vi "CRYSelect curve by name.vi"(9 "Curve name desired (just name, if flat data not wired)":string, 10 "Curve name desired (flat data)":string, 11 "Data array":T2 {"Z data" items=["dB", "Lin"]; "X data" items=["dB", "Lin"]; "Y data" items=["dB", "Lin"]; "Z dB ref" format="%.1f"; "Z axis" items=["Log", "Lin"]; "X dB ref" format="%.1f"; "X axis" items=["Log", "Lin"]; "Y axis" items=["Log", "Lin"]; "Y dB ref" format="%.1f"; "Curve"."z" format="%.2f"; "Curve"."y" format="%.2f"; "Curve"."x" format="%.2f"}) -> (0 "Exists?":bool, 1 "Valid curve desired?":bool, 3 "Desired Curve":T1={"Name"="", "Curve"=[], "X data"=1, "Y data"=1, "Z data"=1, "X axis"=0, "Y axis"=1, "Z axis"=1, "X unit"="Hz", "Y unit"="", "Z unit"="deg.", "X dB ref"=1.0, "Y dB ref"=1.0, "Z dB ref"=1.0, "single val"=FALSE, "protected"=FALSE, "display X"=TRUE, "display Y"=TRUE, "display Z"=TRUE, "Test Info"="", "Step No."=0, "Plot Settings"={"Color"=0, "Interpolation"=0, "Point Style"=0, "Line Style"=0, "Point Color"=0, "Line Width"=0, "Bar Plot Style"=0, "Fill To"=0}, "AutoProtect"=FALSE} {"Z data" items=["dB", "Lin"]; "X data" items=["dB", "Lin"]; "Y data" items=["dB", "Lin"]; "Z dB ref" format="%.1f"; "Z axis" items=["Log", "Lin"]; "X dB ref" format="%.1f"; "X axis" items=["Log", "Lin"]; "Y axis" items=["Log", "Lin"]; "Y dB ref" format="%.1f"; "Curve"."z" format="%.2f"; "Curve"."y" format="%.2f"; "Curve"."x" format="%.2f"}, 5 "index of element":i32)   [LabVIEW 2013]
uses:
  Typedef Control/CRYData Cluster Array.ctl
  Typedef Control/CRYData Cluster.ctl
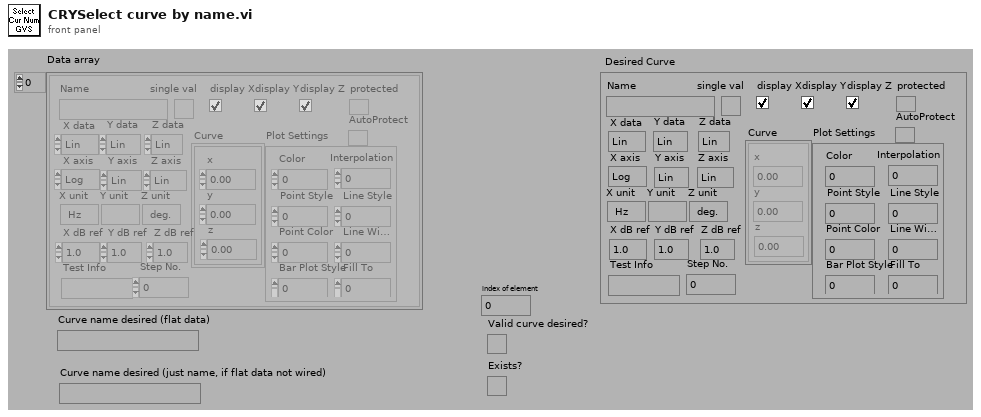
[diagram p1: front panel]
types:
  T1 = typedef "CRYData Cluster.ctl" = cluster{"Name":string, "Curve":cluster{"x":dbl, "y":dbl, "z":dbl}[], "X data":u16, "Y data":u16, "Z data":u16, "X axis":u16, "Y axis":u16, "Z axis":u16, "X unit":string, "Y unit":string, "Z unit":string, "X dB ref":dbl, "Y dB ref":dbl, "Z dB ref":dbl, "single val":bool, "protected":bool, "display X":bool, "display Y":bool, "display Z":bool, "Test Info":string, "Step No.":i32, "Plot Settings":cluster{"Color":u32, "Interpolation":u8, "Point Style":u8, "Line Style":u8, "Point Color":u32, "Line Width":u8, "Bar Plot Style":u8, "Fill To":i16}, "AutoProtect":bool}
  T2 = typedef "CRYData Cluster Array.ctl" = T1[]
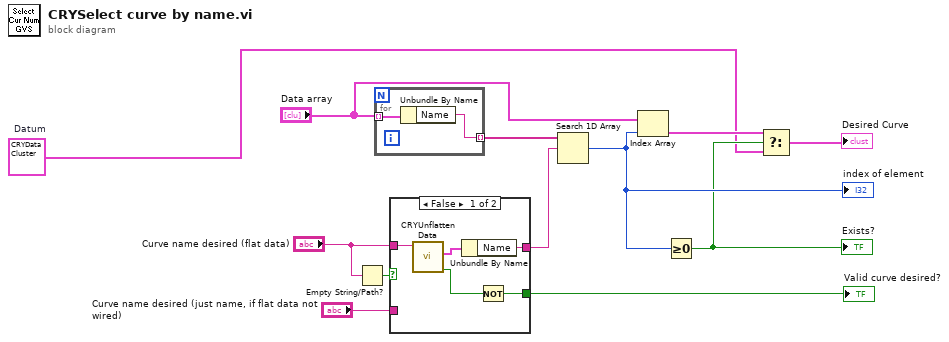
[diagram p0: block diagram]
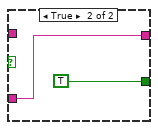
[diagram p2: hidden frame]
diagram:
  w2 = T1 {"Name"="", "Curve"=[], "X data"=1, "Y data"=1, "Z data"=1, "X axis"=0, "Y axis"=1, "Z axis"=1, "X unit"="Hz", "Y unit"="", "Z unit"="deg.", "X dB ref"=1.0, "Y dB ref"=1.0, "Z dB ref"=1.0, "single val"=FALSE, "protected"=FALSE, "display X"=TRUE, "display Y"=TRUE, "display Z"=TRUE, "Test Info"="", "Step No."=0, "Plot Settings"={"Color"=0, "Interpolation"=0, "Point Style"=0, "Line Style"=0, "Point Color"=0, "Line Width"=0, "Bar Plot Style"=0, "Fill To"=0}, "AutoProtect"=FALSE}  # Datum
  n1 = Empty String/Path?(string/path="Curve name desired (flat data)") -> (empty?=w9:bool)
  n2 = for {
    tunnel: "Data array" -> [w14] mode=indexing
    tunnel: [w13] -> w6 mode=indexing
    n3 = Unbundle By Name(w14) -> ("Name"=w13:string)
  }
  n4 = case shown="False" w9 {
    tunnel: "Curve name desired (flat data)" -> [w17 _]
    tunnel: [w19 w21] -> w12
    tunnel: [w18 TRUE] -> w11
    tunnel: "Curve name desired (just name, if flat data not wired)" -> [_ w21]
    frame False {
      n5 = call "CRYUnflatten Data.vi"("Unflatten data"=w17) -> ("Error?"=w15:bool, "Datum"=w16:T1)  [unwired: 9 out]
      n6 = Unbundle By Name(w16) -> ("Name"=w19:string)
      n7 = Not(x=w15) -> (.not. x?=w18:bool)
    }
    frame True {
    }
  }
  "Valid curve desired?" <- w11
  n8 = Search 1D Array(1D array=w6, element=w12) -> (index of element=w5:i32)  [unwired: 1 out]
  "index of element" <- w5
  n9 = Index Array(array="Data array", index=w5) -> (element=w3:T1)
  n10 = Greater Or Equal To 0?(x=w5) -> (x >= 0?=w4:bool)
  "Exists?" <- w4
  n11 = Select(t=w3, s=w4, f=w2) -> (s? t:f=→"Desired Curve":T1)
